vi "channel add to configuration.vi"(6 "channel classification":T1, 8 "error in":errorcluster, 9 "data type":T2, 10 "channel name":string, 11 "shared memory module configuration in":refnum<class "shared memory configuration.lvclass">) -> (0 "error out":errorcluster, 2 "created channel":refnum<class "TBM channel.lvclass">, 3 "shared memory module configuration out":refnum<class "shared memory configuration.lvclass">)   [LabVIEW 2013, in "shared memory configuration.lvclass"]
doc: "***TODO***\n\n<B>Input Parameters</B>\n\n<B>channel classification (output data)</B> ***TODO***channel classification (output data)***enum values: input data,output data,processing parameter,processing result\n\n<B>error in</B> describes error conditions that occur before this node runs. This input provides standard error in functionality.\n\n<B>data type</B> ***TODO***data type***enum values: Double,Single,I64,I32,I16,I8,U64,U32,U16,U8,Boolean,String,Array of Double,Array of Single,Array of I64,Array of I32,Array of I16,Array of I8,Array of U64,Array of U32,Array of U16,Array of U8,Array of Boolean,Array of String\n\n<B>channel name</B> ***TODO***channel name\n\n<B>shared memory module configuration in</B> ***TODO***shared memory module configuration in\n\n<B>Output Parameters</B>\n\n<B>error out</B> contains error information. This output provides standard error out functionality.\n\n<B>created channel</B> ***TODO***created channel\n\n<B>shared memory module configuration out</B> ***TODO***shared memory module configuration out"
uses:
  shared memory configuration.lvclass
  <vilib>/NI/Tag Bus/tag/Data Type.ctl
  <vilib>/NI/Tag Bus Module Framework/channel/TBM channel.lvclass
  <vilib>/NI/Tag Bus Module Framework/channel/channel classification.ctl
  shared memory configuration.lvclass/shared memory configuration.ctl
  Line.ctl
  <vilib>/NI/Tag Bus/tag/tag descriptor.lvclass
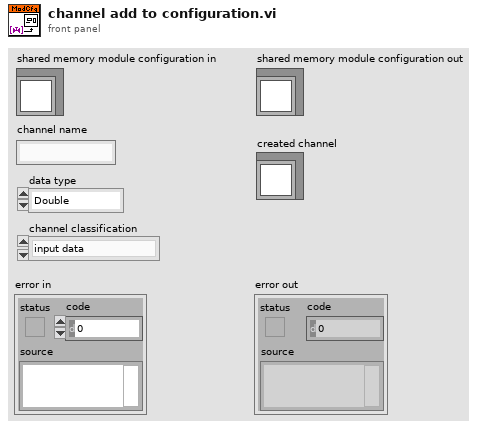
[diagram p1: front panel]
types:
  T1 = typedef "TBM channel.lvclass/channel classification.ctl" = enum16{"input data", "output data", "processing parameter", "processing result"}
  T2 = typedef "tag bus.lvlib/tag descriptor.lvclass/Data Type.ctl" = enum16{"Double", "Single", "I64", "I32", "I16", "I8", "U64", "U32", "U16", "U8", "Boolean", "String", "Array of Double", "Array of Single", "Array of I64", "Array of I32", "Array of I16", "Array of I8", "Array of U64", "Array of U32", "Array of U16", "Array of U8", "Array of Boolean", "Array of String"}
  T3 = typedef "shared memory configuration.lvclass/Line.ctl" = cluster{"name":string, "data type":T2, "channel":refnum<class "TBM channel.lvclass">}
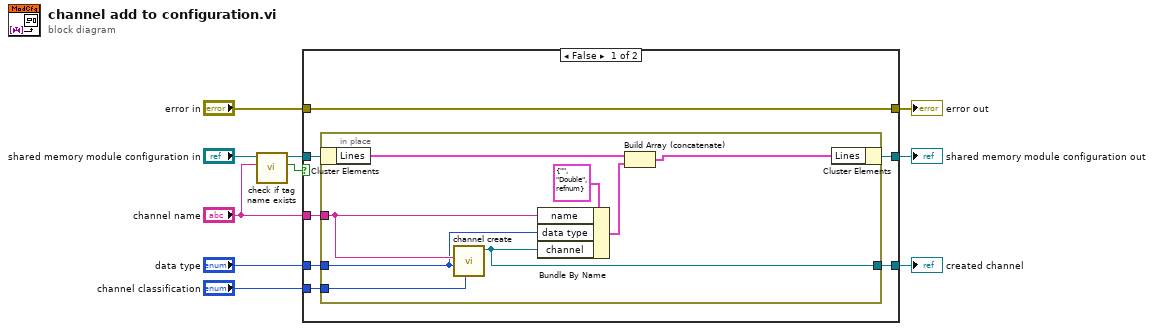
[diagram p0: block diagram]
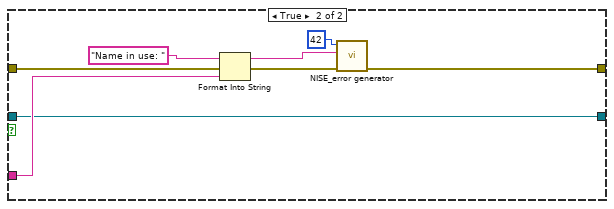
[diagram p2: hidden frame]
diagram:
  n1 = call "check if tag name exists.vi"("name to locate"="channel name", "shared memory module configuration in"="shared memory module configuration in") -> ("found?"=w7:bool, "shared memory module configuration out"=w5:refnum<class "shared memory configuration.lvclass">)  [unwired: 6 in, 2 out]
  n2 = case shown="False" w7 {
    tunnel: [w15 w32] -> w9
    tunnel: "error in" -> [w15 w33]
    tunnel: "channel name" -> [w14 w28]
    tunnel: [w16 w26] -> w6
    tunnel: w5 -> [w17 w26]
    tunnel: "data type" -> [w13 _]
    tunnel: [w12 _] -> w2
    tunnel: "channel classification" -> [w11 _]
    frame False {
      n3 = in-place {
        in-place-border: w14 -> [w21]
        in-place-border: w13 -> [w20]
        in-place-border: [w18] -> w12
        in-place-border: w11 -> [w19]
        n4 = in-place-cluster #1(w17) -> ("Lines"=w25:T3[])
        n5 = call "channel create.vi"("channel classification (output data)"=w19, "data type"=w20, "channel name"=w21) -> ("channel"=w18:refnum<class "TBM channel.lvclass">)  [unwired: 8 in]
        n6 = Bundle By Name(cluster=T3 {"name"="", "data type"=enum."Double", "channel"=refnum} ("alarm config"), "name"=w21, "data type"=w20, "channel"=w18) -> (w22:T3)
        n7 = Build Array (concatenate)(w25, w22) -> (w24:T3[])
        n8 = in-place-cluster #1("Lines"=w24) -> (w16:refnum<class "shared memory configuration.lvclass">)
      }
    }
    frame True {
      n9 = Format Into String(initial string="Name in use: " ("append error message"), error in=w33, w28) -> (resulting string=w27:string, error out=w30:errorcluster)  [unwired: 1 in]
      n10 = call <vilib>:"NISE_error generator.vi"("error in"=w30, "append error message"=w27, "error code (0)"=42) -> ("error out"=w32:errorcluster)  [unwired: 6 in]
    }
  }
  "error out" <- w9
  "shared memory module configuration out" <- w6
  "created channel" <- w2
